vi "tm_closecamera.vi"(8 "error in (no error)":errorcluster, 11 "Handle in":u32) -> (0 "error out":errorcluster)   [LabVIEW 2015]
uses:
  tmcamcon.dll
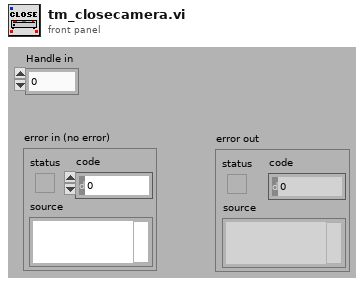
[diagram p1: front panel]
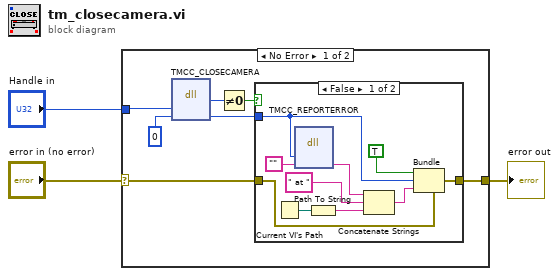
[diagram p0: block diagram]
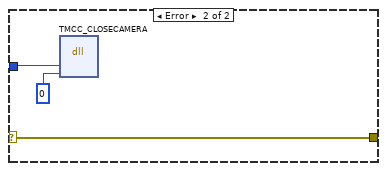
[diagram p3: hidden frame]
diagram:
  n1 = case shown="No Error" "error in (no error)" {
    selector: "error in (no error)" -> [w6 w22]
    tunnel: [w4 w22] -> w2
    tunnel: "Handle in" -> [w8 w23]
    frame No Error {
      n2 = dll-call lib="tmcamcon.dll" fn="TMCC_CLOSECAMERA"("index"=w8, "Erval"=0) -> (w10:u32, "Erval"=w7:i32)  [unwired: 4 in, 2 out]
      n3 = Not Equal To 0?(x=w10) -> (x != 0?=w5:bool)
      n4 = case shown="False" w5 {
        tunnel: w6 -> [w20 w21]
        tunnel: [w19 w21] -> w4
        tunnel: w7 -> [w13 _]
        frame False {
          n5 = Current VI's Path() -> (path=w18:path)
          n6 = dll-call lib="tmcamcon.dll" fn="TMCC_REPORTERROR"("error"=w13, "buf"="") -> ("buf"=w12:string)  [unwired: 5 in, 2 out]
          n7 = Path To String(path=w18) -> (string=w14:string)
          n8 = Concatenate Strings(w12, " at ", w14) -> (w17:string)
          n9 = Bundle(cluster=w20, "status"=TRUE, "code"=w13, "source"=w17) -> (w19:errorcluster)
        }
        frame True {
        }
      }
    }
    frame Error {
      n10 = dll-call lib="tmcamcon.dll" fn="TMCC_CLOSECAMERA"("HDCAM"=w23, "Erval"=0) -> ()  [unwired: 6 in, 2 out]
    }
  }
  "error out" <- w2
